vi "Lookup Drag Data.vi"(10 "Name":string, 11 "Data":T1(array[cluster])) -> (2 "Found":bool, 3 "Value":variant)   [LabVIEW 2020, in "VolatusGUIEditor.lvlib" / "Editor.lvclass"]
uses:
  Editor.lvclass
  Editor.lvclass/Editor.ctl
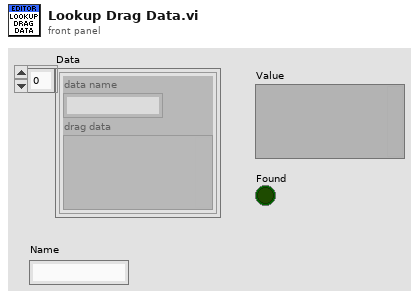
[diagram p1: front panel]
types:
  T1 = cluster{"data name":string, "drag data":variant}[]
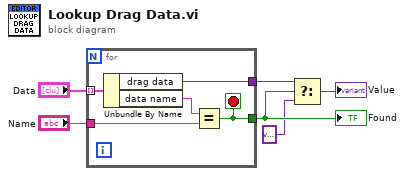
[diagram p0: block diagram]
diagram:
  n1 = for {
    tunnel: "Data" -> [w11] mode=indexing
    tunnel: [w10] -> w4
    tunnel: "Name" -> [w9]
    tunnel: [w7] -> w3
    stop <- w7 stop-if-true
    n2 = Unbundle By Name(w11) -> ("drag data"=w10:variant, "data name"=w8:string)
    n3 = Equal?(x=w8, y=w9) -> (x = y?=w7:bool)
  }
  "Found" <- w3
  n4 = Select(t=w4, s=w3, f=variant) -> (s? t:f=→"Value":variant)
